vi "sv_Check for f0 Change.vi"(8 "error in (no error)":errorcluster, 11 "power spectrum":cluster{"f0":dbl, "df":dbl, "Spectrum":dbl[]} {"Spectrum" format="%.2f"; "df" format="%.2f"; "f0" format="%.2f"}) -> (0 "error out":errorcluster, 1 "parameter has changed":bool, 3 "dup power spectrum":cluster{"f0":dbl, "df":dbl, "Spectrum":dbl[]} {"Spectrum" format="%.2f"; "df" format="%.2f"; "f0" format="%.2f"})   [LabVIEW 2017]
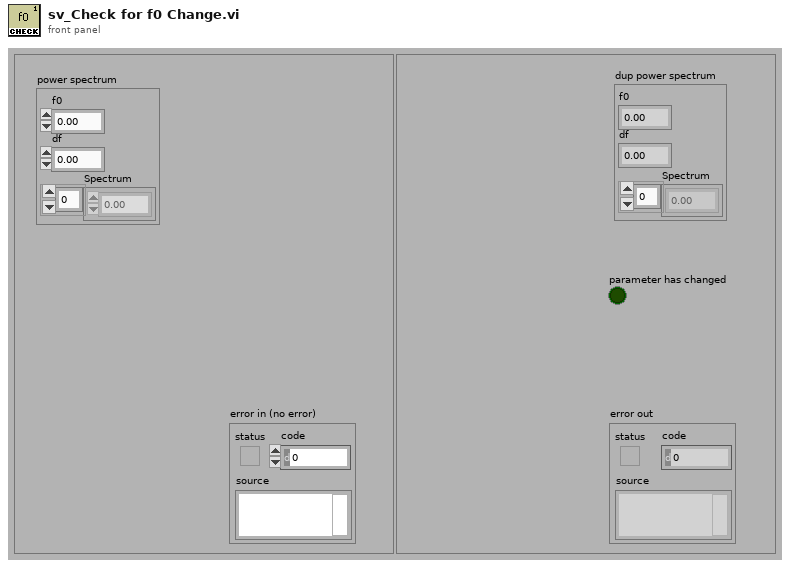
[diagram p1: front panel]
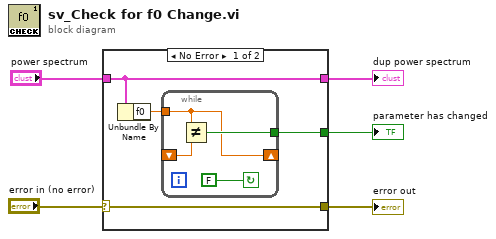
[diagram p0: block diagram]
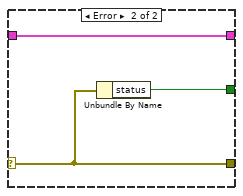
[diagram p2: hidden frame]
diagram:
  n1 = case shown="No Error" "error in (no error)" {
    selector: "error in (no error)" -> [w8 w15]
    tunnel: "power spectrum" -> [w7 w16]
    tunnel: [w8 w15] -> w4
    tunnel: [w7 w16] -> w3
    tunnel: [w6 w14] -> w1
    frame No Error {
      n2 = Unbundle By Name(w7) -> ("f0"=w9:dbl)
      n3 = while {
        tunnel: [w12] -> w6
        tunnel: w9 -> [w10]
        shift-left: _ -> [w11]
        shift-right: [w10] -> _
        stop <- FALSE continue-if-true
        n4 = Not Equal?(x=w10, y=w11) -> (x != y?=w12:bool)
      }
    }
    frame Error {
      n5 = Unbundle By Name(w15) -> ("status"=w14:bool)
    }
  }
  "error out" <- w4
  "dup power spectrum" <- w3
  "parameter has changed" <- w1
